vi "update XY graph axes test.vi"() -> ()   [LabVIEW 2016]
uses:
  <vilib>/Platform/TimedLoop/XDataNode/timing_clust.ctl
  <vilib>/Platform/TimedLoop/XDataNode/nitl_modes.ctl
  <vilib>/Platform/TimedLoop/XDataNode/wakeup.ctl
  <vilib>/platform/TimedLoop/XDataNode/XDataNode.xnode
  <vilib>/Platform/TimedLoop/XDataNode/XDNodeRunTimeDep.lvlib
panel:
  in  "y":u16(ring) items=["a", "b", "c", "d", "e"]
  in  "x":u16(ring) items=["a", "b", "c", "d", "e"]
  out "xy Cluster":cluster{dbl[], dbl[]}
  out "Cluster":T1
  out "e":dbl
  out "d":dbl
  out "c":dbl
  out "b":dbl
  out "a":dbl
  out "N of For Loop":i32
  in  "N of For Loop":i32
  out "Timed Loop Index":i32
  out "For Loop Index":i32
  out "XY Graph":cluster{dbl[], dbl[]}(graph)
  in  "stop":bool
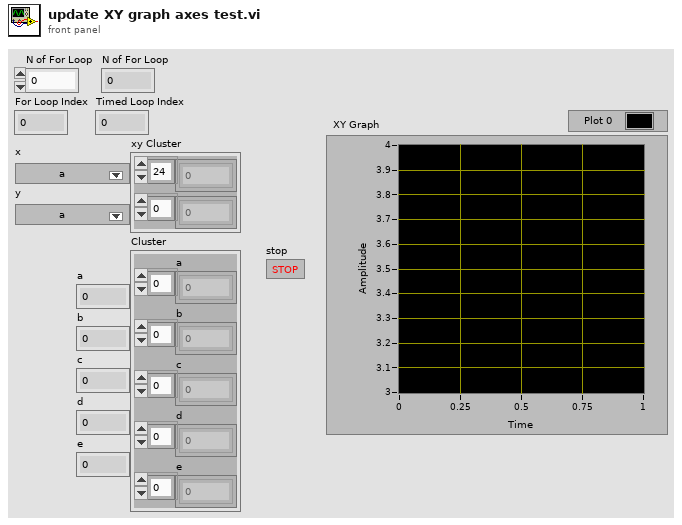
[diagram p1: front panel]
types:
  T1 = cluster{"a":dbl[], "b":dbl[], "c":dbl[], "d":dbl[], "e":dbl[]}
  T2 = typedef "XDNodeRunTimeDep.lvlib/timing_clust.ctl" = cluster{"Expected End [f-1]":u64, "Actual End [f-1]":u64, "Finished Late? [f-1]":bool, "Expected End [i-1]":u64, "Actual End [i-1]":u64, "Finished Late? [i-1]":bool, "Expected Start [i]":u64, "Actual Start [i]":u64, "Expected Start [f]":u64, "Actual Start [f]":u64, "Source Name":string, "Structure Name":string, "Period":i64, "Deadline":i64, "Offset":i64, "Start":i64, "Priority":i32, "Timeout":i32, "Mode":T3, "Wakeup Reason":T4, "Error":errorcluster, "Source Type":string, "Secondary Source Type":string, "Global End Time":u64, "Global Start Time":u64, "Frame Duration":u64, "Iteration Duration":u64, "Assigned CPU":i32, "I/O Scan Engine Mode":u32}
  T3 = typedef "XDNodeRunTimeDep.lvlib/nitl_modes.ctl" = enum32{"No Change", "Process missed periods, maintain original phase", "Discard missed periods, maintain original phase", "Process missed periods, ignore original phase", "Discard missed periods, ignore original phase"}
  T4 = typedef "XDNodeRunTimeDep.lvlib/wakeup.ctl" = enum32{"Normal", "Aborted", "Asynchronous wakeup", "Timing source error", "Timed loop error", "Timeout"}
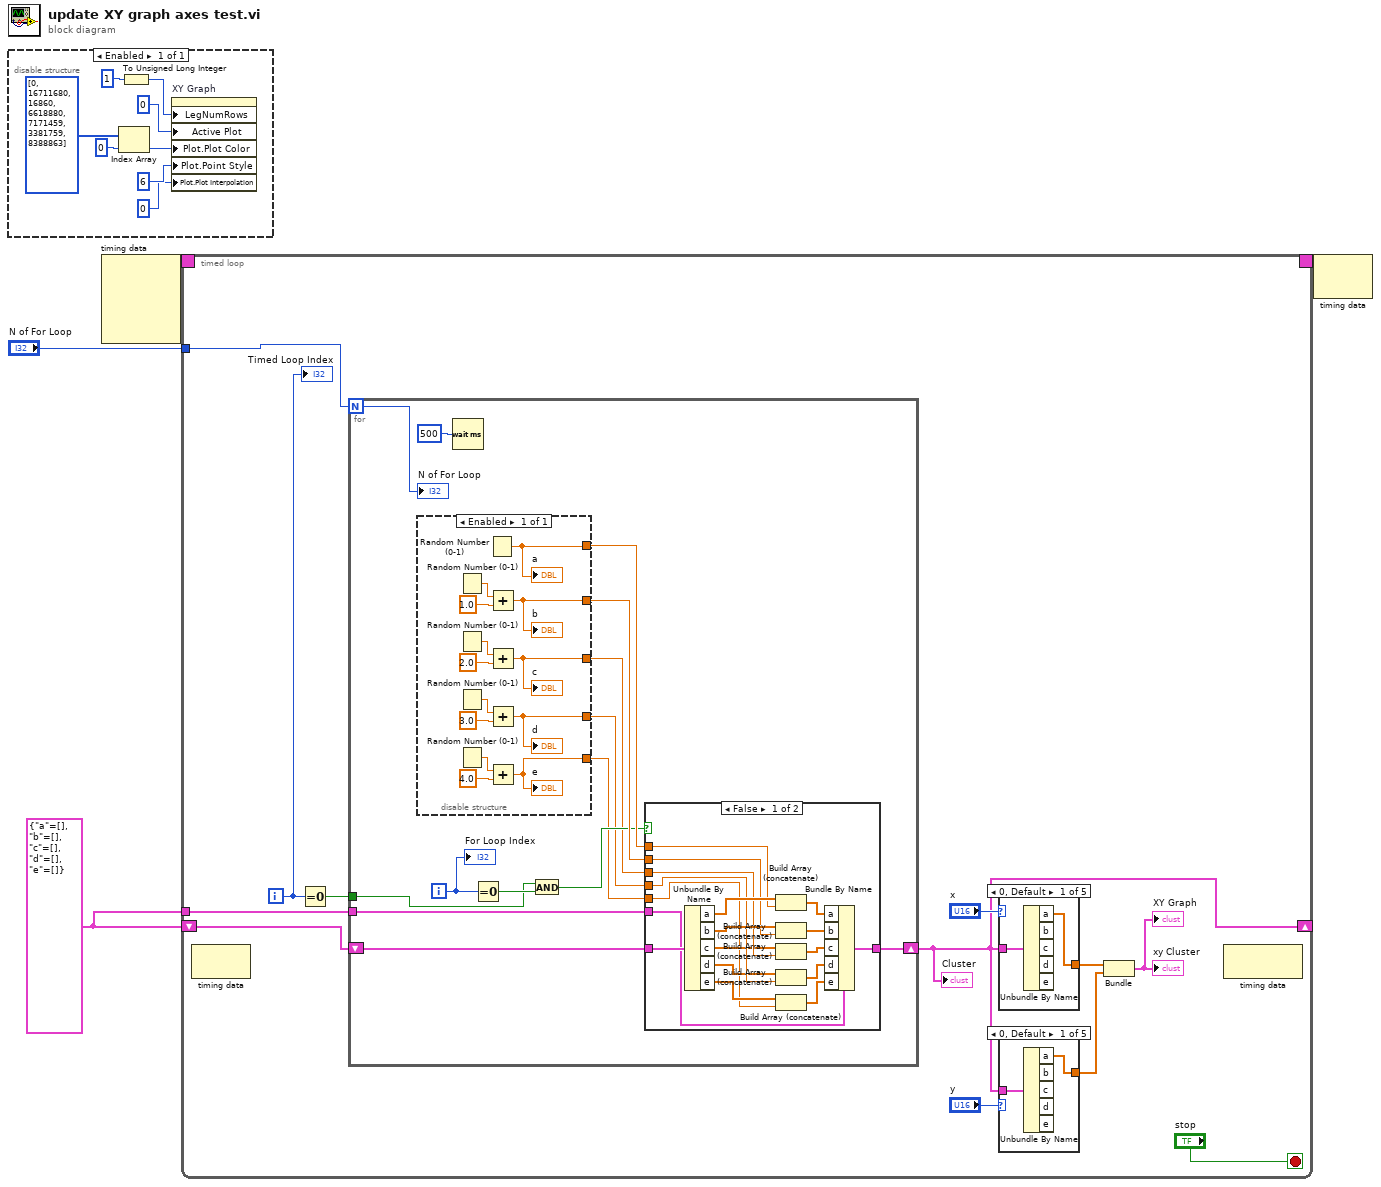
[diagram p0: block diagram]
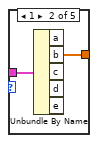
[diagram p2: hidden frame]
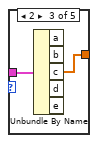
[diagram p3: hidden frame]
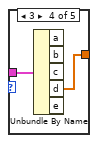
[diagram p4: hidden frame]
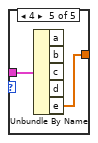
[diagram p5: hidden frame]
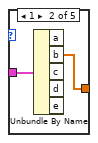
[diagram p6: hidden frame]
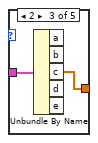
[diagram p7: hidden frame]
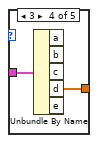
[diagram p8: hidden frame]
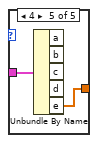
[diagram p9: hidden frame]
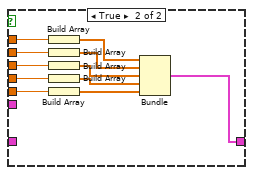
[diagram p10: hidden frame]
diagram:
  w1 = T1 {"a"=[], "b"=[], "c"=[], "d"=[], "e"=[]}
  n1 = disable-structure shown="Enabled" {
    frame Enabled {
      n2 = Index Array(array=u32[] [0, 16711680, 16860, 6618880, 7171459, 3381759, 8388863], index=0) -> (element=w10:u32)
      n3 = To Unsigned Long Integer(number=1 ("dimension size")) -> (unsigned 32bit integer=w7:u32)
      n4 = property on="XY Graph" class="XYGraph (strict)"("LegNumRows"=w7, "Active Plot"=u32 0, "Plot.Plot Color"=w10, "Plot.Point Style"=u8 6, "Plot.Plot Interpolation"=u8 0) -> ()  [unwired: 2 in, 2 out]
    }
  }
  n5 = node-c288() -> (w4:T2)  [unwired: 4 in]
  n6 = timed-loop {
    timing: w4 -> [_]
    timing-out: [_] -> w3
    shift-right: [w15] -> _
    shift-left: w1 -> [w22]
    tunnel: "N of For Loop" -> [w21]
    tunnel: w1 -> [w19]
    i -> [w23]
    stop <- "stop" stop-if-true
    n7 = node-c288() -> ()  [unwired: 1 in, 1 out]
    n8 = Equal To 0?(x=w23) -> (x = 0?=w20:bool)
    n9 = for {
      N: w21 -> [w53]
      shift-right: [w51] -> w15
      shift-left: w22 -> [w58]
      tunnel: w20 -> [w52]
      tunnel: w19 -> [w47]
      i -> [w56]
      n10 = disable-structure shown="Enabled" {
        disable-tunnel: [w73] -> w60
        disable-tunnel: [w61] -> w59
        disable-tunnel: [w62] -> w50
        disable-tunnel: [w63] -> w49
        disable-tunnel: [w64] -> w48
        frame Enabled {
          n11 = Random Number (0-1)() -> (number: 0 to 1=w69:dbl)
          n12 = Random Number (0-1)() -> (number: 0 to 1=w70:dbl)
          n13 = Random Number (0-1)() -> (number: 0 to 1=w71:dbl)
          n14 = Random Number (0-1)() -> (number: 0 to 1=w72:dbl)
          n15 = Random Number (0-1)() -> (number: 0 to 1=w73:dbl)
          "a" <- w73
          n16 = Add(x=w69, y=1.0) -> (x+y=w61:dbl)
          "b" <- w61
          n17 = Add(x=w70, y=2.0) -> (x+y=w62:dbl)
          "c" <- w62
          n18 = Add(x=w71, y=3.0) -> (x+y=w63:dbl)
          "d" <- w63
          n19 = Add(x=w72, y=4.0) -> (x+y=w64:dbl)
          "e" <- w64
        }
      }
      n20 = Wait (ms)(milliseconds to wait=u32 500) -> ()  [unwired: 1 out]
      n21 = Equal To 0?(x=w56) -> (x = 0?=w57:bool)
      n22 = And(x=w52, y=w57) -> (x .and. y?=w55:bool)
      n23 = case shown="False" w55 {
        tunnel: [w89 w98] -> w51
        tunnel: w58 -> [w88 _]
        tunnel: w59 -> [w86 w99]
        tunnel: w60 -> [w87 w100]
        tunnel: w50 -> [w79 w92]
        tunnel: w49 -> [w78 w93]
        tunnel: w48 -> [w75 w94]
        tunnel: w47 -> [w74 _]
        frame False {
          n24 = Unbundle By Name(w88) -> ("a"=w90:dbl[], "b"=w91:dbl[], "c"=w76:dbl[], "d"=w77:dbl[], "e"=w80:dbl[])
          n25 = Build Array (concatenate)(w90, w87) -> (w85:dbl[])
          n26 = Build Array (concatenate)(w91, w86) -> (w84:dbl[])
          n27 = Build Array (concatenate)(w76, w79) -> (w83:dbl[])
          n28 = Build Array (concatenate)(w77, w78) -> (w82:dbl[])
          n29 = Build Array (concatenate)(w80, w75) -> (w81:dbl[])
          n30 = Bundle By Name(cluster=w74, "a"=w85, "b"=w84, "c"=w83, "d"=w82, "e"=w81) -> (w89:T1)
        }
        frame True {
          n31 = Build Array(w100) -> (w101:dbl[])
          n32 = Build Array(w99) -> (w102:dbl[])
          n33 = Build Array(w92) -> (w97:dbl[])
          n34 = Build Array(w93) -> (w96:dbl[])
          n35 = Build Array(w94) -> (w95:dbl[])
          n36 = Bundle(w101, w102, w97, w96, w95) -> (w98:cluster{dbl[], dbl[], dbl[], dbl[], dbl[]})  [unwired: 1 in]
        }
      }
      "For Loop Index" <- w56
      "N of For Loop" <- w53
    }
    "Cluster" <- w15
    n37 = case shown="0, Default" "x" {
      tunnel: w15 -> [w36 w38 w40 w42 w44]
      tunnel: [w35 w37 w39 w41 w43] -> w18
      frame 0, Default {
        n38 = Unbundle By Name(w36) -> ("a"=w35:dbl[])  [unwired: 4 out]
      }
      frame 1 {
        n39 = Unbundle By Name(w38) -> ("b"=w37:dbl[])  [unwired: 4 out]
      }
      frame 2 {
        n40 = Unbundle By Name(w40) -> ("c"=w39:dbl[])  [unwired: 4 out]
      }
      frame 3 {
        n41 = Unbundle By Name(w42) -> ("d"=w41:dbl[])  [unwired: 4 out]
      }
      frame 4 {
        n42 = Unbundle By Name(w44) -> ("e"=w43:dbl[])  [unwired: 4 out]
      }
    }
    n43 = case shown="0, Default" "y" {
      tunnel: w15 -> [w26 w28 w30 w32 w34]
      tunnel: [w25 w27 w29 w31 w33] -> w13
      frame 0, Default {
        n44 = Unbundle By Name(w26) -> ("a"=w25:dbl[])  [unwired: 4 out]
      }
      frame 1 {
        n45 = Unbundle By Name(w28) -> ("b"=w27:dbl[])  [unwired: 4 out]
      }
      frame 2 {
        n46 = Unbundle By Name(w30) -> ("c"=w29:dbl[])  [unwired: 4 out]
      }
      frame 3 {
        n47 = Unbundle By Name(w32) -> ("d"=w31:dbl[])  [unwired: 4 out]
      }
      frame 4 {
        n48 = Unbundle By Name(w34) -> ("e"=w33:dbl[])  [unwired: 4 out]
      }
    }
    n49 = Bundle("e"=w18, "e"=w13) -> (→"XY Graph" →"xy Cluster":cluster{"e":dbl[], "e":dbl[]})  [unwired: 1 in]
    n50 = node-c288() -> ()  [unwired: 1 in, 1 out]
    "Timed Loop Index" <- w23
  }
  n51 = node-c288(w3) -> ()  [unwired: 1 out]
